vi "Initialization.vi"(8 "error in (no error)":errorcluster, 10 "port":u16=8082, 11 "TcpIpProc in":refnum<class "TcpIpProc.lvclass">) -> (0 "error out":errorcluster, 3 "TcpIpProc out":refnum<class "TcpIpProc.lvclass">)   [LabVIEW 2024, in "TCPIPActor.lvlib" / "TcpIpProc.lvclass"]
uses:
  TcpIpProc.lvclass
  TcpIpProc.lvclass/TcpIpProc.ctl
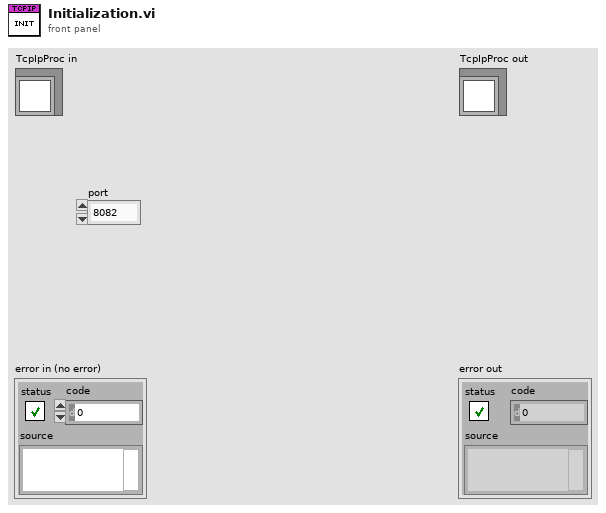
[diagram p1: front panel]
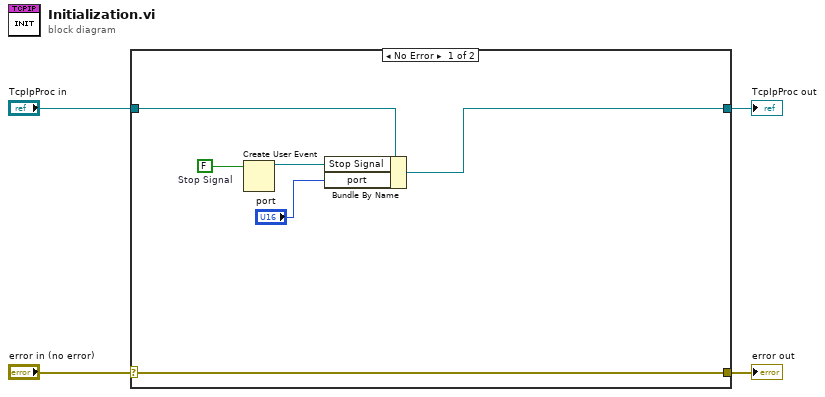
[diagram p0: block diagram]
diagram:
  n1 = case shown="No Error" "error in (no error)" {
    selector: "error in (no error)" -> [w10 w12]
    tunnel: [w10 w12] -> w3
    tunnel: [w6 w11] -> w1
    tunnel: "TcpIpProc in" -> [w7 w11]
    frame No Error {
      w9 = FALSE  # Stop Signal
      n2 = Create User Event(user event datatype=w9) -> (user event=w8:refnum<user-event>)  [unwired: 1 in, 1 out]
      n3 = Bundle By Name(cluster=w7, "Stop Signal"=w8, "port"="port") -> (w6:refnum<class "TcpIpProc.lvclass">)
    }
    frame Error {
    }
  }
  "error out" <- w3
  "TcpIpProc out" <- w1
